vi "diming light as water pump.vi"(3 "LED Channel (digital)":u8=9, 9 "PWM Out (0-1)":dbl(knob) scale=0.0..1.0 scale format="%.2f", 11 "Serial Port":refnum<visa-resource-name>="COM9") -> ()   [LabVIEW 2020]
doc: "Manually blink and LED attached to a digital output channel of a LINX device by clicking and LED control in LabVIEW."
uses:
  <vilib>/MakerHub/LINX/Public/Peripherals/PWM/PWM Set Duty Cycle 1 Chan.vi
  <vilib>/MakerHub/LINX/Public/Utilities/Open Serial.vi
  <vilib>/MakerHub/LINX/Public/Peripherals/PWM/PWM Set Duty Cycle N Chans.vi
  <vilib>/MakerHub/LINX/LMH-LINX.lvlib
panel:
  out "Loop Rate (Hz)":u32=69
  in  "Stop Button":bool
  # "This example was created by combining code from LINX - Blink (Simple), LINX - PWM 1 Channel, and LINX - Photocell VIs\nIn addition, the circuitry for how to control a DC motor was modified from the example in:\nElegoo The Most Complete Starter Kit for UNO V2.0.2020.4.3\\English\\Part 2 Module Learning\\2.23 DC Motors"
  # "LINX Device Settings"
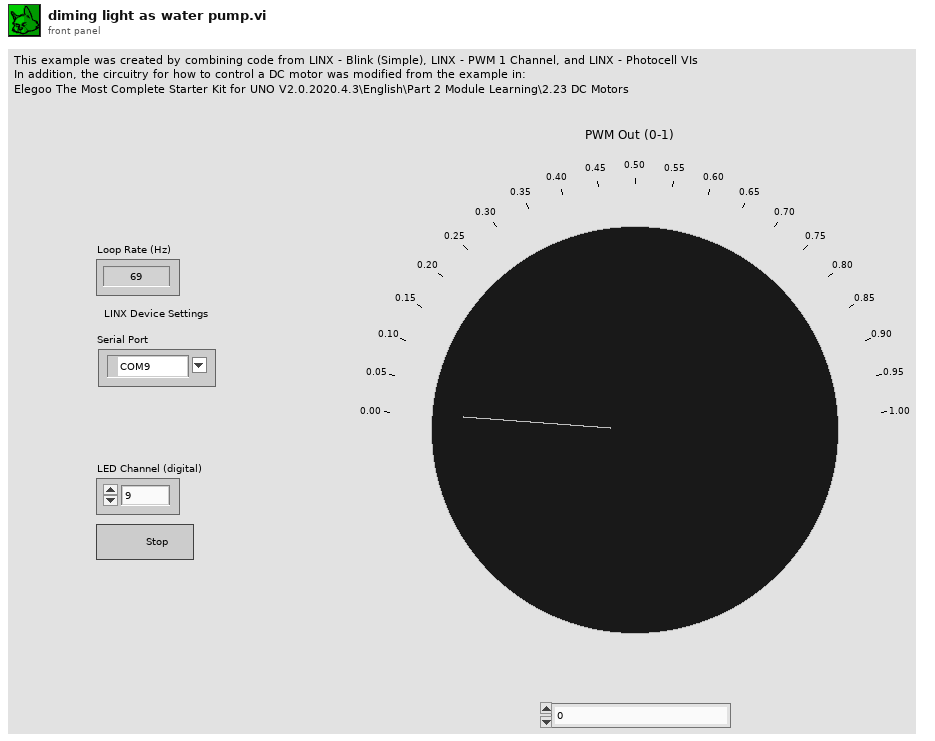
[diagram p1: front panel]
types:
  T1 = typedef "LMH-LINX.lvlib/LINX Ref.ctl" = cluster{"IO":T2, "Interface":T3, "LINX Device Config":T4}
  T2 = typedef "LMH-LINX.lvlib/Platform.ctl" = enum16{"Remote", "Local"}
  T3 = typedef "LMH-LINX.lvlib/Interface.ctl" = enum16{"Serial", "TCP"}
  T4 = typedef "LMH-LINX.lvlib/Device.lvlib/LINX Device Config.ctl" = cluster{"Interface":T3, "COM Port":refnum<visa-resource-name>, "TCP Configuration":T5, "Device Family":u8, "Device ID":u8, "Device Name":string, "TCP Ref":refnum<k5>, "Channels":T6}
  T5 = typedef "LMH-LINX.lvlib/Device.lvlib/TCP Config.ctl" = cluster{"IP Address":string, "Port":u16}
  T6 = typedef "LMH-LINX.lvlib/Channels.ctl" = cluster{"DI":u8[], "DO":u8[], "AI":u8[], "AO":u8[], "PWM":u8[], "QE":u8[], "UART":u8[], "I2C 2":u8[], "SPI":u8[], "CAN":u8[], "Servo":u8[], "AI Ref (V)":dbl, "AI Resolution (Bits)":u8, "AO Ref (V)":dbl, "AO Resolution (Bits)":u8}
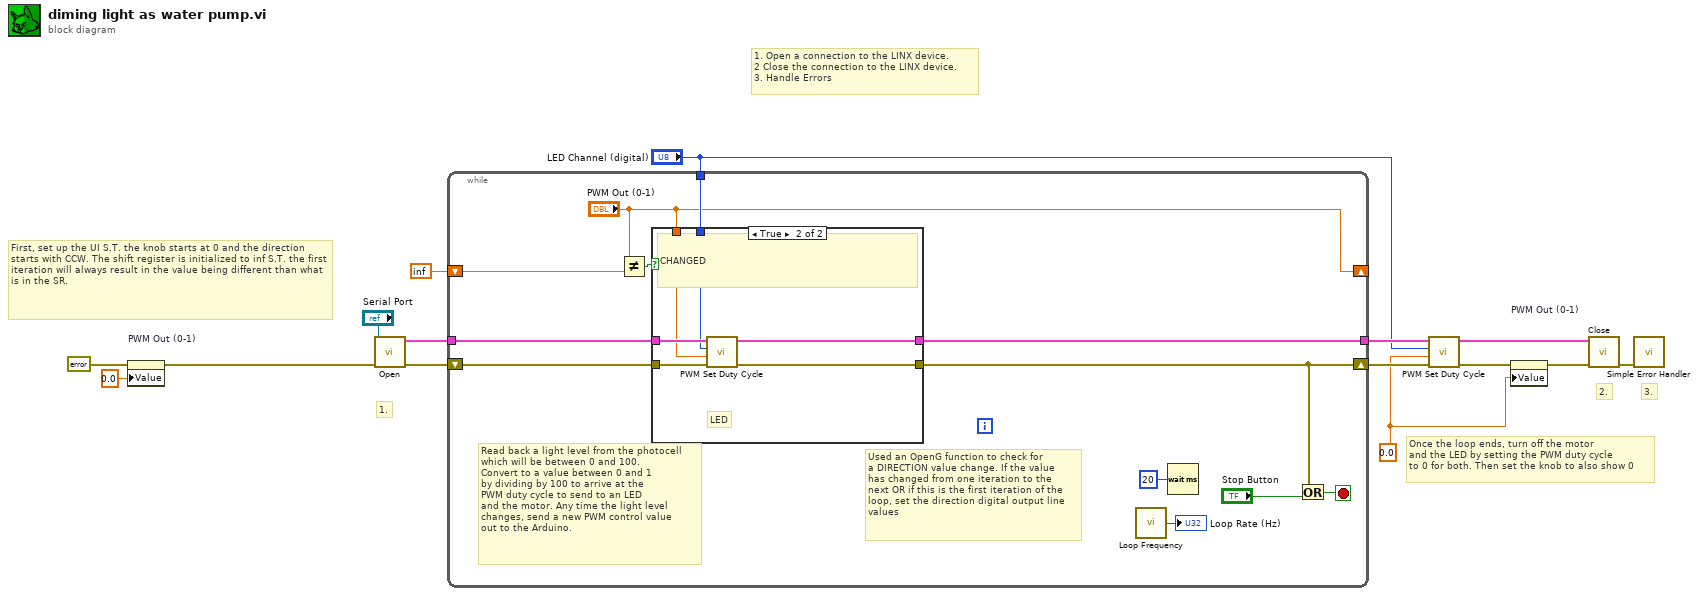
[diagram p0: block diagram]
diagram:
  w5 = 0.0
  # "Once the loop ends, turn off the motor\nand the LED by setting the PWM duty cycle\nto 0 for both. Then set the knob to also show 0"
  # "First, set up the UI S.T. the knob starts at 0 and the direction starts with CCW. The shift register is initialized to inf S.T. the first iteration will always result in the value being different than what is in the SR."
  # "1. Open a connection to the LINX device.\n2 Close the connection to the LINX device.\n3. Handle Errors"
  # "3."
  # "2."
  # "1."
  n1 = property on="PWM Out (0-1)" class="Knob (strict)"(error in=errorcluster {"status"=FALSE, "code"=0, "source"=""} ("Error In"), "Value"=0.0) -> (error out=w1:errorcluster)  [unwired: 1 in, 1 out]
  n2 = call-poly <vilib>:"Open.vi"("Error In"=w1, "Serial Port"="Serial Port") -> ("Error Out"=w14:errorcluster, "LINX Resource"=w15:T1)  [unwired: 7 in, 1 out]
  n3 = while {
    tunnel: w15 -> [w17]
    tunnel: [w19] -> w7
    shift-right: [w20] -> w8
    shift-left: w14 -> [w16]
    tunnel: "LED Channel (digital)" -> [w24]
    shift-right: ["PWM Out (0-1)"] -> _
    shift-left: inf -> [w23]
    stop <- w27 stop-if-true
    # "Used an OpenG function to check for\na DIRECTION value change. If the value\nhas changed from one iteration to the\nnext OR if this is the first iteration of the\nloop, set the direction digital output line\nvalues"
    # "Read back a light level from the photocell\nwhich will be between 0 and 100.\nConvert to a value between 0 and 1\nby dividing by 100 to arrive at the\nPWM duty cycle to send to an LED\nand the motor. Any time the light level\nchanges, send a new PWM control value\nout to the Arduino."
    n4 = Not Equal?(x="PWM Out (0-1)", y=w23) -> (x != y?=w22:bool)
    n5 = case shown="True" w22 {
      tunnel: w17 -> [w29 w35]
      tunnel: [w29 w31] -> w19
      tunnel: w16 -> [w28 w34]
      tunnel: [w28 w30] -> w20
      tunnel: "PWM Out (0-1)" -> [_ w32]
      tunnel: w24 -> [_ w33]
      frame False {
        # "SAME"
      }
      frame True {
        # "LED"
        # "CHANGED"
        n6 = call-poly <vilib>:"PWM Set Duty Cycle.vi"("Error In"=w34, "Duty Cycle (0-1)"=w32, "PWM Channel"=w33, "LINX Resource"=w35) -> ("Error Out"=w30:errorcluster, "LINX Resource"=w31:T1)  [unwired: 6 in]
      }
    }
    n7 = call <vilib>:"Loop Frequency.vi"() -> ("Loop Rate (Hz)"=→"Loop Rate (Hz)":u32)
    n8 = Wait (ms)(milliseconds to wait=u32 20) -> ()  [unwired: 1 out]
    n9 = Or(x=w20, y="Stop Button") -> (x .or. y?=w27:bool)
  }
  n10 = call-poly <vilib>:"PWM Set Duty Cycle.vi"("Error In"=w8, "Duty Cycle (0-1)"=w5, "PWM Channel"="LED Channel (digital)", "LINX Resource"=w7) -> ("Error Out"=w2:errorcluster, "LINX Resource"=w4:T1)  [unwired: 6 in]
  n11 = property on="PWM Out (0-1)" class="Knob (strict)"(error in=w2, "Value"=w5) -> (error out=w3:errorcluster)  [unwired: 1 in, 1 out]
  n12 = call <vilib>:"Close.vi"("Error In"=w3, "LINX Resource"=w4) -> ("Error Out"=w12:errorcluster)  [unwired: 9 in]
  n13 = call <vilib>:"Simple Error Handler.vi"("error in (no error)"=w12) -> ()  [unwired: 4 in, 5 out]
